vi "Mass Dispense Control (SubVI).vi"(0 "Weight (Grams)":dbl, 1 "Dispense Setpoint (%)":dbl=2.0, 2 "Fill Setpoint (g)":dbl=1000.0, 3 "Settings":T2={"ON Settings"={"Enable Dynamic Setpoint?"=TRUE, "Enable Dynamic Dispense Time?"=TRUE, "Enable Drain Rate Functions"=TRUE, "Dispense Sample Time (s)"=0.5, "Dispense Slope Ave"=0, "ON Timeout (sec)"=600.0, "1st Setpoint (% of Target)"=0.0, "2nd Setpoint (% of Target)"=0.0, "3rd Setpoint (% of Target)"=0.0, "Measure Dispense Delay (sec)"=0.0, "Settle Slope Sample Time (s)"=0.0}, "OFF Settings"={"Drain Sample Time (s)"=0.5, "Drain Rate Ave Size"=5, "Drain Rate Limits (± g/sec)"=10.0, "Level Slope Range (± g/sec)"=0.25, "OFF Timeout (sec)"=0.0, "Near SP Slope Level (± g/sec)"=0.01, "Near Setpoint Threshold (%)"=95.0}, "Overshoot Settings"={"Time Limit (s)"=60.0, "Container MAX (g)"=1500.0, "Max FILL Slope (+/- g/sec)"=10.0, "% Overshot to Enable (>)"=0.25}, "FILL Timeout (s)"=300.0, "Full Settle Time (s)"=20.0, "Pre-Hydrate \nSpray Time (s)"=10.0, "Pre-Hydrate \nWait Time (s)"=30.0}, 4 "Product Weight (g)":dbl, 5 "Overshoot Adjust?":bool=TRUE, 6 "STOP Dispense":bool, 8 "START Dispense":bool) -> (11 "Spray Count":i32, 14 "Signals":T4, 16 "Values":T5 {"Drain Time (s)" format="%.2f"; "Drain Rate (g/sec)" format="%.2f"; "Time Elapsed (s)" format="%.2f"; "Time Target (s)" format="%.2f"; "Dynamic Setpoint (g)" format="%.2f"; "Static Setpoint (g)" format="%.2f"; "Grams to Setpoint" format="%.2f"; "Adjusted Mass (g)" format="%.2f"; "Dispense Rate (g/sec)" format="%.2f"; "Fill Mass (g)" format="%.2f"; "Fill Rate (g/sec)" format="%.2f"}, 17 "Product Values":T1, 18 "Hydration (g)":dbl, 19 "Dispense Mode":T3(ring))   [LabVIEW 2009]
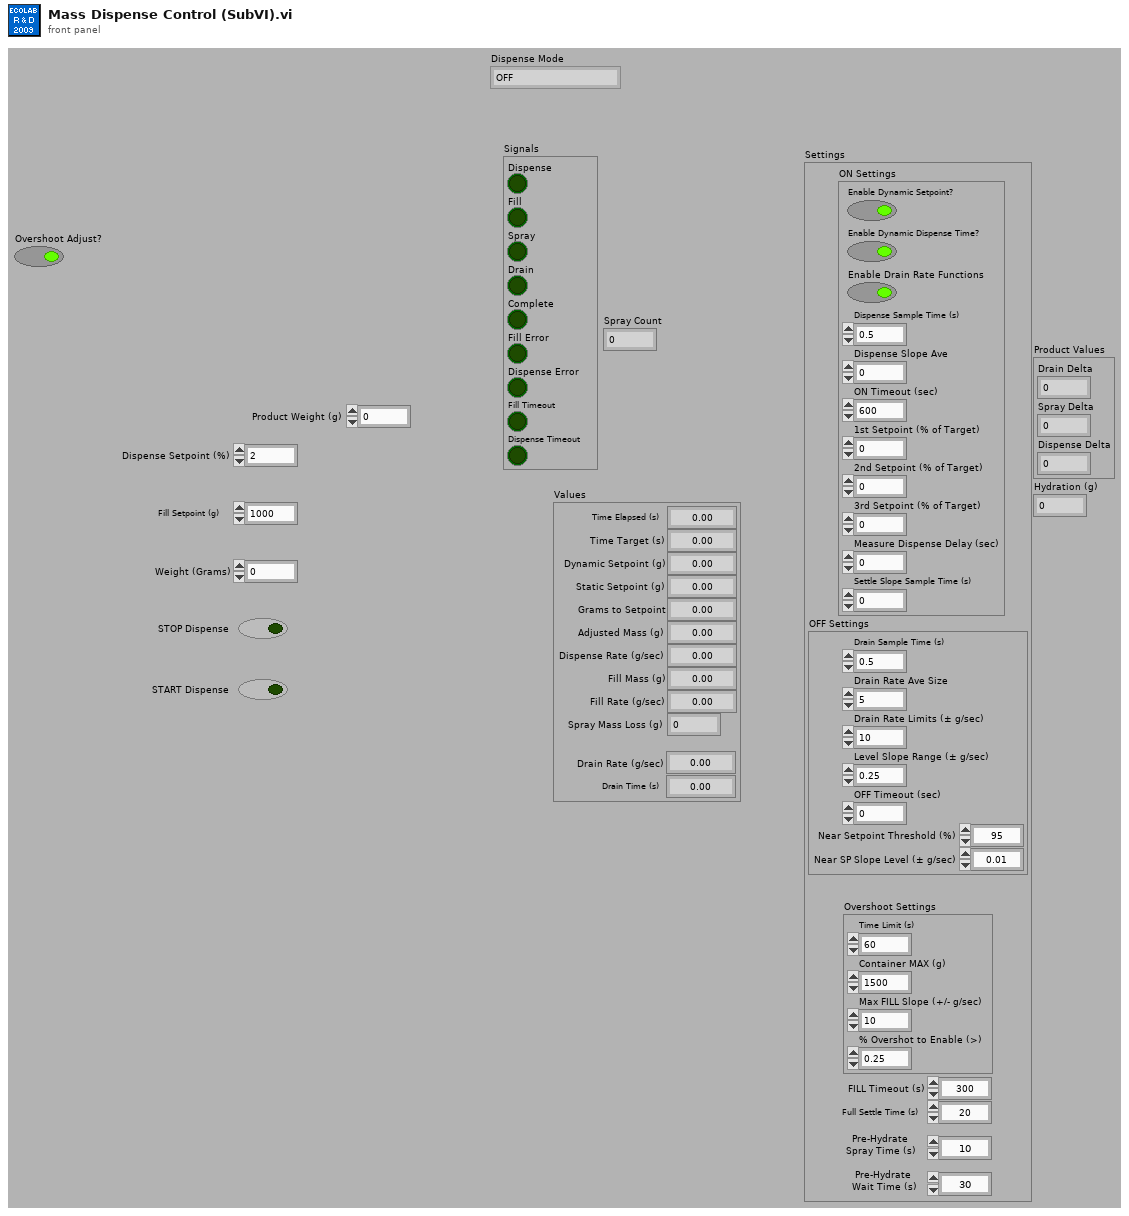
[diagram p1: front panel]
types:
  T1 = cluster{"Drain Delta":dbl, "Spray Delta":dbl, "Dispense Delta":dbl}
  T2 = cluster{"ON Settings":cluster{"Enable Dynamic Setpoint?":bool, "Enable Dynamic Dispense Time?":bool, "Enable Drain Rate Functions":bool, "Dispense Sample Time (s)":dbl, "Dispense Slope Ave":i32, "ON Timeout (sec)":dbl, "1st Setpoint (% of Target)":dbl, "2nd Setpoint (% of Target)":dbl, "3rd Setpoint (% of Target)":dbl, "Measure Dispense Delay (sec)":dbl, "Settle Slope Sample Time (s)":dbl}, "OFF Settings":cluster{"Drain Sample Time (s)":dbl, "Drain Rate Ave Size":i32, "Drain Rate Limits (± g/sec)":dbl, "Level Slope Range (± g/sec)":dbl, "OFF Timeout (sec)":dbl, "Near SP Slope Level (± g/sec)":dbl, "Near Setpoint Threshold (%)":dbl}, "Overshoot Settings":cluster{"Time Limit (s)":dbl, "Container MAX (g)":dbl, "Max FILL Slope (+/- g/sec)":dbl, "% Overshot to Enable (>)":dbl}, "FILL Timeout (s)":dbl, "Full Settle Time (s)":dbl, "Pre-Hydrate \nSpray Time (s)":dbl, "Pre-Hydrate \nWait Time (s)":dbl}
  T3 = enum16{"OFF", "INITIAL", "FILL", "DISPENSE", "ADJUST"}
  T4 = cluster{"Dispense":bool, "Fill":bool, "Spray":bool, "Drain":bool, "Complete":bool, "Fill Error":bool, "Dispense Error":bool, "Fill Timeout":bool, "Dispense Timeout":bool}
  T5 = cluster{"Time Elapsed (s)":dbl, "Time Target (s)":dbl, "Dynamic Setpoint (g)":dbl, "Static Setpoint (g)":dbl, "Grams to Setpoint":dbl, "Adjusted Mass (g)":dbl, "Dispense Rate (g/sec)":dbl, "Fill Mass (g)":dbl, "Fill Rate (g/sec)":dbl, "Spray Mass Loss (g)":dbl, "Drain Rate (g/sec)":dbl, "Drain Time (s)":dbl}
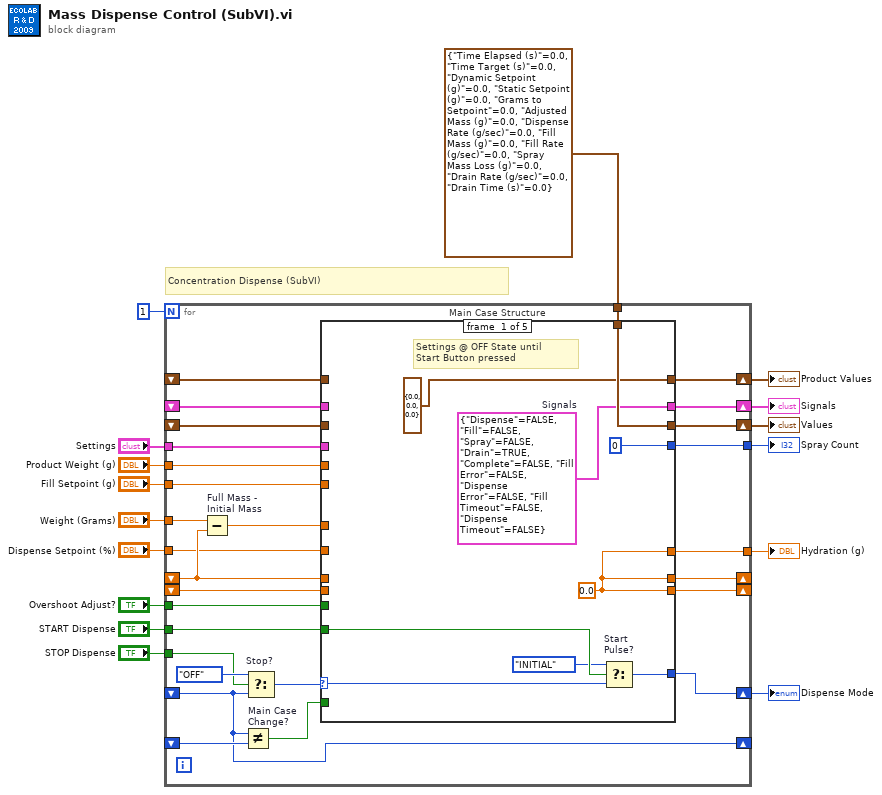
[diagram p0: block diagram]
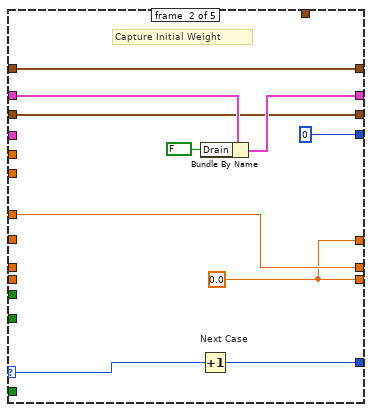
[diagram p2: hidden frame]
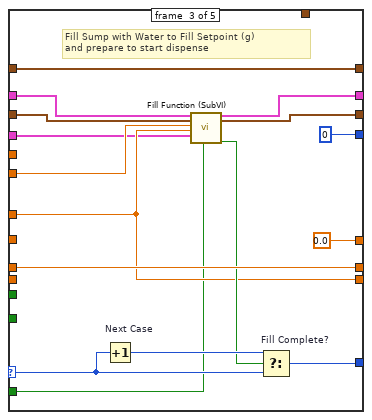
[diagram p3: hidden frame]
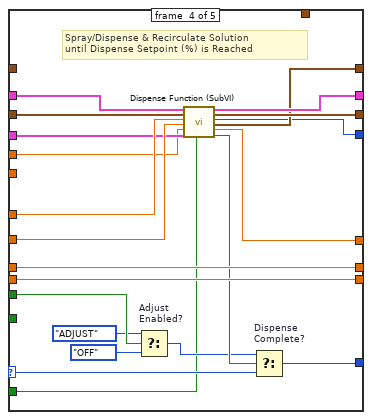
[diagram p4: hidden frame]
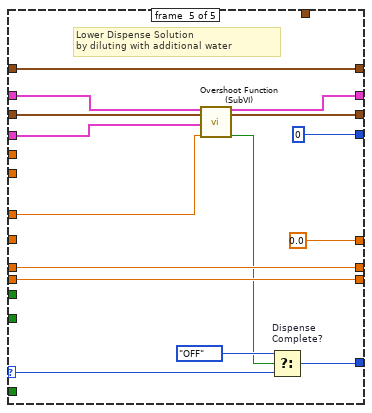
[diagram p5: hidden frame]
diagram:
  # "Concentration Dispense (SubVI)"
  n1 = for {
    N: 1 -> [_]
    tunnel: "Weight (Grams)" -> [w37]
    shift-right: [w44] -> w6
    shift-left: _ -> [w18]
    tunnel: "Fill Setpoint (g)" -> [w32]
    tunnel: "Dispense Setpoint (%)" -> [w28]
    shift-right: [w43] -> w8
    shift-left: _ -> [w33]
    shift-right: [w42] -> _
    shift-left: _ -> [w38]
    tunnel: "START Dispense" -> [w41]
    tunnel: "STOP Dispense" -> [w39]
    shift-right: [w36] -> _
    shift-left: _ -> [w35]
    tunnel: "Settings" -> [w27]
    tunnel: T5 {"Time Elapsed (s)"=0.0, "Time Target (s)"=0.0, "Dynamic Setpoint (g)"=0.0, "Static Setpoint (g)"=0.0, "Grams to Setpoint"=0.0, "Adjusted Mass (g)"=0.0, "Dispense Rate (g/sec)"=0.0, "Fill Mass (g)"=0.0, "Fill Rate (g/sec)"=0.0, "Spray Mass Loss (g)"=0.0, "Drain Rate (g/sec)"=0.0, "Drain Time (s)"=0.0} -> [w31]
    shift-right: [w30] -> w9
    shift-left: _ -> [w29]
    tunnel: "Overshoot Adjust?" -> [w26]
    tunnel: "Product Weight (g)" -> [w25]
    shift-right: [w24] -> w3
    shift-left: _ -> [w23]
    tunnel: [w22] -> w2
    shift-right: [w18] -> _
    shift-left: _ -> [w21]
    tunnel: [w17] -> w1
    n2 = Subtract "Full Mass -\nInitial Mass"(x=w37, y=w38) -> (x-y=w34:dbl)
    n3 = Not Equal? "Main Case\nChange?"(x=w18, y=w21) -> (x != y?=w19:bool)
    n4 = Select "Stop?"(t=T3."OFF" ("Mode (Read)"), s=w39, f=w18) -> (s? t:f=w20:T3)
    n5 = case "Main Case Structure" shown="\"DISPENSE\"" w20 {
      selector: w20 -> [w52 w63 w78 w97 w106]
      tunnel: w34 -> [_ w62 w72 w91 w104]
      tunnel: [w51 w61 w77 w100 w108] -> w44
      tunnel: w32 -> [_ _ w75 _ _]
      tunnel: [w49 w59 w71 w95 w112] -> w43
      tunnel: w33 -> [_ w60 w74 w96 w113]
      tunnel: [w46 w62 w76 w99 w115] -> w42
      tunnel: w38 -> [_ _ w76 w99 w115]
      tunnel: w41 -> [w53 _ _ _ _]
      tunnel: [w46 w55 w72 w98 w114] -> w36
      tunnel: w35 -> [_ _ _ w98 w114]
      tunnel: w31 -> [w50 _ _ _ _]
      tunnel: [w50 w57 w69 w92 w110] -> w30
      tunnel: w29 -> [_ w57 w70 w94 w111]
      tunnel: w28 -> [_ _ _ w90 _]
      tunnel: w27 -> [_ _ w66 w85 w105]
      tunnel: w26 -> [_ _ _ w89 _]
      tunnel: w25 -> [_ _ _ w84 _]
      tunnel: [T1 {"Drain Delta"=0.0, "Spray Delta"=0.0, "Dispense Delta"=0.0} ("Product Values") w56 w68 w83 w103] -> w24
      tunnel: w23 -> [_ w56 w68 _ w103]
      tunnel: [w46 w55 0.0 ("Hydration (g)") w82 0.0 ("Hydration (g)")] -> w22
      tunnel: w19 -> [_ _ w65 w81 _]
      tunnel: [0 ("Spray Count") 0 ("Spray Count") 0 ("Spray Count") w80 0 ("Spray Count")] -> w17
      frame #0 {
        w49 = T4 {"Dispense"=FALSE, "Fill"=FALSE, "Spray"=FALSE, "Drain"=TRUE, "Complete"=FALSE, "Fill Error"=FALSE, "Dispense Error"=FALSE, "Fill Timeout"=FALSE, "Dispense Timeout"=FALSE}  # Signals
        w46 = 0.0 ("Weight (Grams)")
        # "Settings @ OFF State until\nStart Button pressed"
        n6 = Select "Start\nPulse?"(t=T3."INITIAL" ("Mode (Read)"), s=w53, f=w52) -> (s? t:f=w51:T3)
      }
      frame #1 {
        w55 = 0.0 ("Weight (Grams)")
        # "Capture Initial Weight"
        n7 = Increment "Next Case"(x=w63) -> (x+1=w61:T3)
        n8 = Bundle By Name(cluster=w60, "Drain"=FALSE) -> (w59:T4)
      }
      frame #2 {
        # "Fill Sump with Water to Fill Setpoint (g)\nand prepare to start dispense"
        n9 = Increment "Next Case"(x=w78) -> (x+1=w79:T3)
        n10 = call "Fill Function (SubVI).vi"("Signals IN"=w74, "Values IN"=w70, "FILL Setpoint (g)"=w75, "Measured Mass (g)"=w72, "Settings"=w66, "Main Case Change?"=w65) -> ("Signals OUT"=w71:T4, "Values OUT"=w69:T5, "Fill FN Complete"=w73:bool)  [unwired: 1 in, 10 out]
        n11 = Select "Fill Complete?"(t=w79, s=w73, f=w78) -> (s? t:f=w77:T3)
      }
      frame #3 {
        # "Spray/Dispense & Recirculate Solution\nuntil Dispense Setpoint (%) is Reached"
        n12 = Select "Adjust\nEnabled?"(t=T3."ADJUST" ("Mode (Read)"), s=w89, f=T3."OFF" ("Mode (Read)")) -> (s? t:f=w86:T3)
        n13 = call "Dispense Function (SubVI).vi"("Signals IN"=w96, "Values IN"=w94, "Measured Mass (g)"=w91, "Main Concentration Setpoint (%)"=w90, "Product Weight (g)"=w84, "Settings"=w85, "Main Case Change?"=w81) -> ("Signals OUT"=w95:T4, "Values OUT"=w92:T5, "Spray Count"=w80:i32, "Product Values"=w83:T1, "Hydration (g)"=w82:dbl, "Dispense Complete?"=w93:bool)  [unwired: 7 out]
        n14 = Select "Dispense\nComplete?"(t=w86, s=w93, f=w97) -> (s? t:f=w100:T3)
      }
      frame #4 {
        # "Lower Dispense Solution\nby diluting with additional water"
        n15 = call "Overshoot Function (SubVI).vi"("Signals IN"=w113, "Values IN"=w111, "Settings"=w105, "Measured Mass (g)"=w104) -> ("Signals OUT"=w112:T4, "Values OUT"=w110:T5, "Complete"=w107:bool)  [unwired: 4 in, 9 out]
        n16 = Select "Dispense\nComplete?"(t=T3."OFF" ("Mode (Read)"), s=w107, f=w106) -> (s? t:f=w108:T3)
      }
    }
  }
  "Values" <- w9
  "Signals" <- w8
  "Dispense Mode" <- w6
  "Product Values" <- w3
  "Hydration (g)" <- w2
  "Spray Count" <- w1
